vi "EditServerChannelInteractive.vi"() -> ()   [LabVIEW 2022 SP3]
uses:
  Sub VIs/ADAM Controls/Ch_description_ADAM.ctl
  Sub VIs/ADAM Controls/Module_type_ADAM.ctl
  Sub VIs/ADAM Controls/Function_ADAM.ctl
  Sub VIs/ADAM Controls/Channel_State.ctl
  Sub VIs/ADAM Controls/Calib_type_ADAM.ctl
  Sub VIs/ADAM Controls/Address.ctl
  Sub VIs/ADAM Controls/Channel_names.ctl
  EditServerChannelInteractive.ctl
  ADAM Server/ADAM_Global.vi
panel:
  in  "showFP":bool
  in  "chsOff":bool
  in  "chsOn":bool
  out "NewVal":i32[](array[numeric])
  in  "Set Value":dbl
  in  "channelTypes":T1
  in  "Channel Select":i32[](listbox)
  in  "stop":bool
  in  "reloadChannels":bool
  in  "deleteChannel":bool
  in  "reloadDescription":bool
  in  "updateChDescription":bool
  in  "updateValue":bool
  out "Message":string
  out "Value":dbl
  out "String":string
  out "Help":string
  in  "Search String":string
  in  "Ch Description":T2={"Ch Name"="", "Type"="", "Function"=enum."Analogue Input", "Ch State"=enum."On", "Calibration type"="", "A"=0.0, "B"=0.0, "C"=0.0, "D"=0.0, "Comments"="", "Address"={"Main"=0, "Ch."=0, "Sub"=0, "Port Name"=""}, "String"="", "Duty"=65535} {"Duty" format="%016b"; "D" format="%#_5g"; "C" format="%#_5g"; "B" format="%#_5g"; "A" format="%#_5g"}
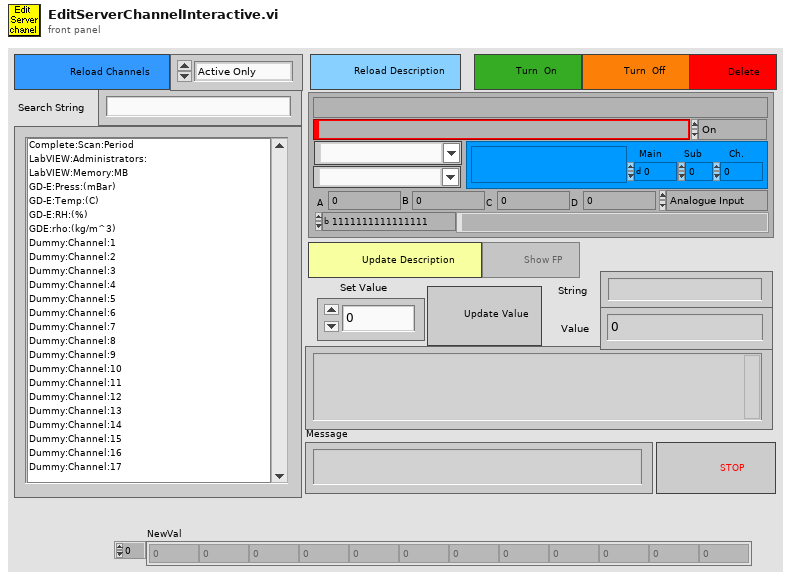
[diagram p1: front panel]
types:
  T1 = typedef "Channel_names.ctl" = enum16{"Active Only", "Active + Off", "All Channels", "Changeable Only", "Always Off", "Always On", "Always Off or On"}
  T2 = typedef "Ch_description_ADAM.ctl" = cluster{"Ch Name":string, "Type":T3, "Function":T4, "Ch State":T5, "Calibration type":T6, "A":dbl, "B":dbl, "C":dbl, "D":dbl, "Comments":string, "Address":T7, "String":string, "Duty":u16}
  T3 = typedef "Module_type_ADAM.ctl" = string
  T4 = typedef "Function_ADAM.ctl" = enum16{"Analogue Input", "Digital Input", "Event counter", "Event rate", "Analogue Output", "Digital Output", "Relay Output"}
  T5 = typedef "Channel_State.ctl" = enum16{"On", "Off", "Always On", "Always Off"}
  T6 = typedef "Calib_type_ADAM.ctl" = string
  T7 = typedef "Address.ctl" = cluster{"Main":i32, "Ch.":i32, "Sub":i32, "Port Name":string}
  T8 = typedef "EditServerChannelInteractive.ctl" = enum16{"Start", "Wait for user", "Check Channels", "Get Channel Names", "Get Current Value", "Get Channel Description", "Update Channel Value", "Update Channel State", "Update Channel Description", "Delete Channel", "Multi Channel", "openFP"}
  T9 = enum8{"Enabled", "Disabled", "Disabled and Grayed Out"}
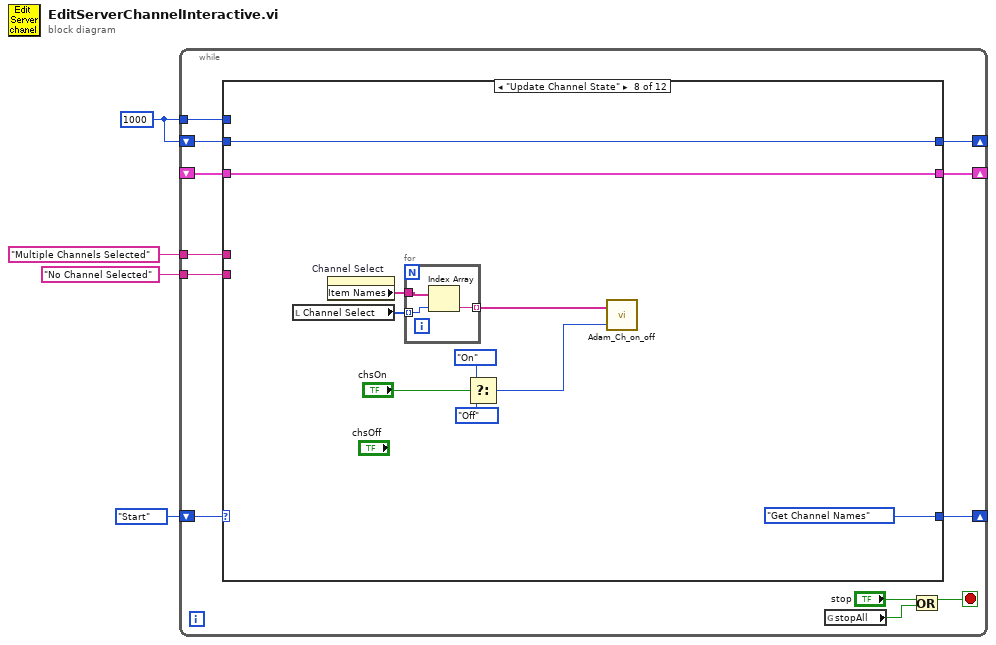
[diagram p0: block diagram]
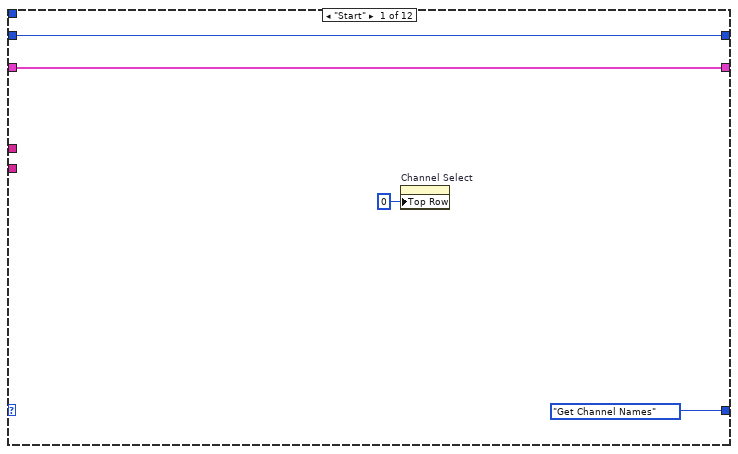
[diagram p2: hidden frame]
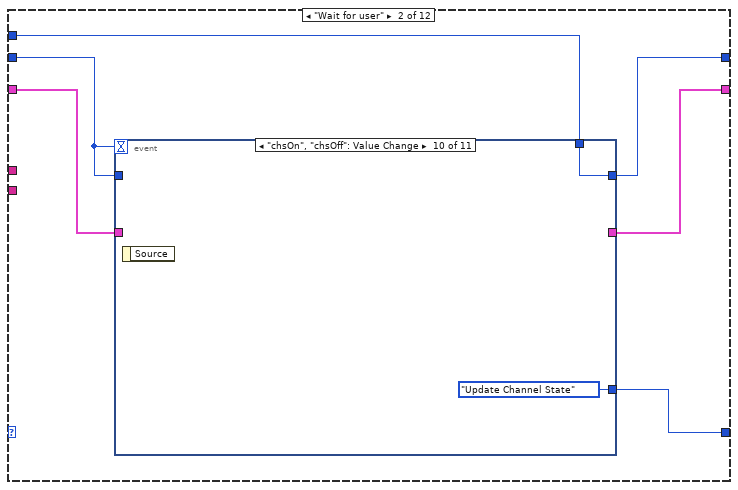
[diagram p3: hidden frame]
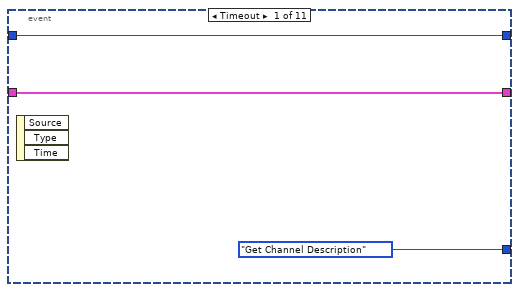
[diagram p4: hidden frame]
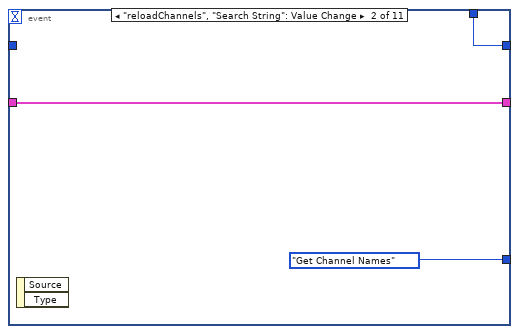
[diagram p5: hidden frame]
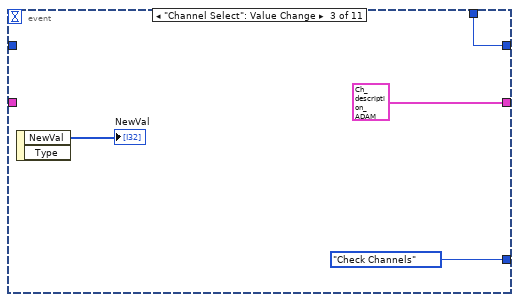
[diagram p6: hidden frame]
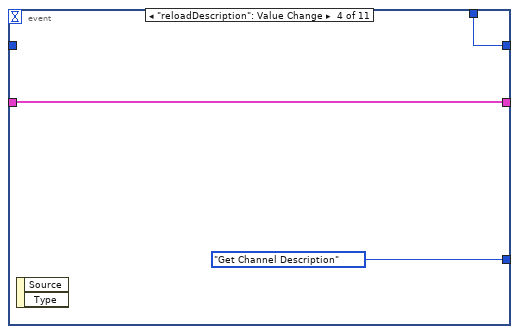
[diagram p7: hidden frame]
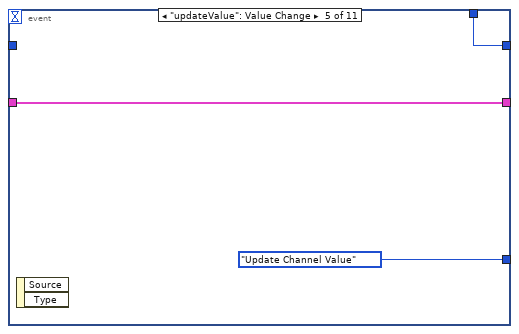
[diagram p8: hidden frame]
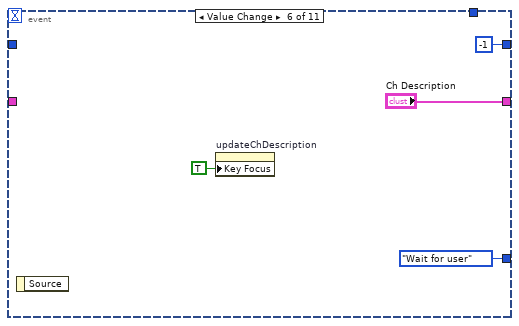
[diagram p9: hidden frame]
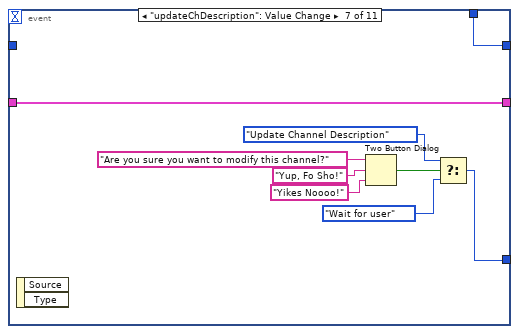
[diagram p10: hidden frame]
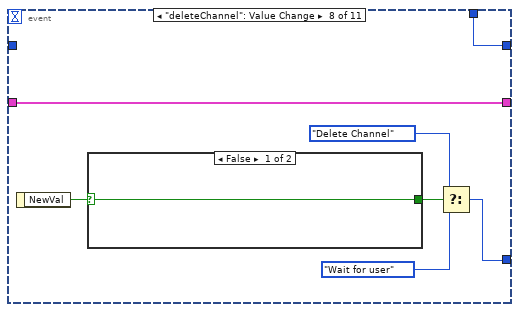
[diagram p11: hidden frame]
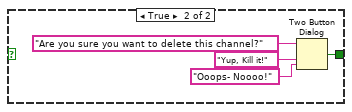
[diagram p12: hidden frame]
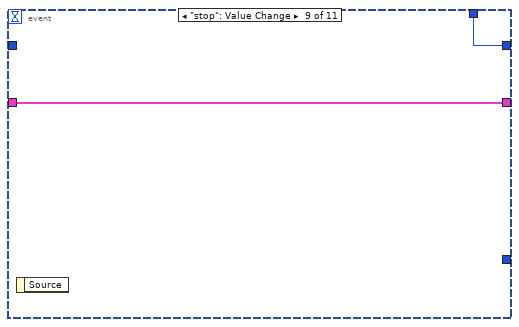
[diagram p13: hidden frame]
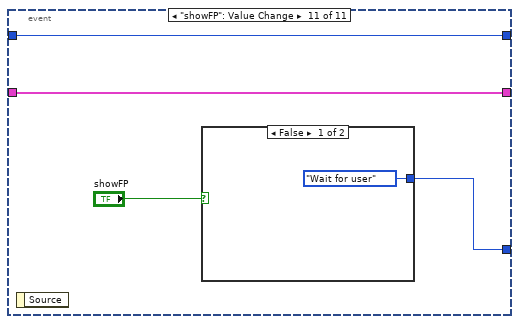
[diagram p14: hidden frame]
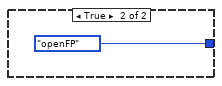
[diagram p15: hidden frame]
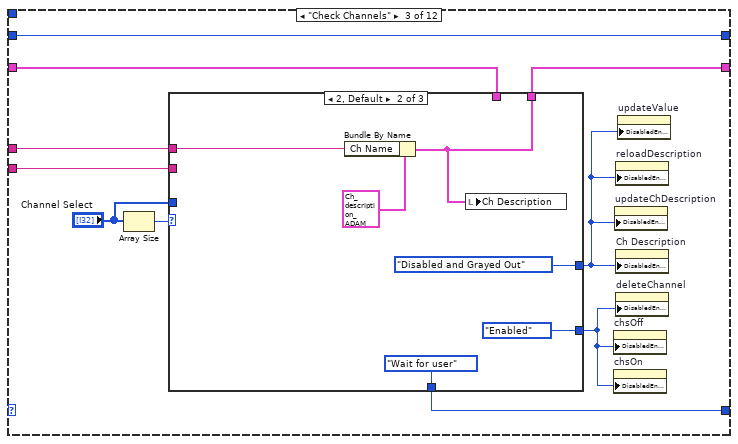
[diagram p16: hidden frame]
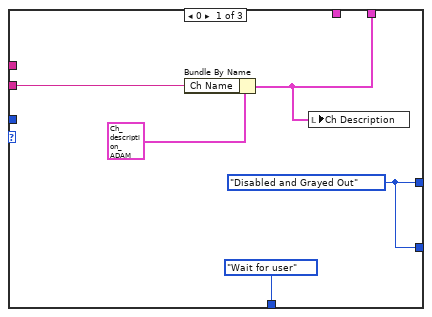
[diagram p17: hidden frame]
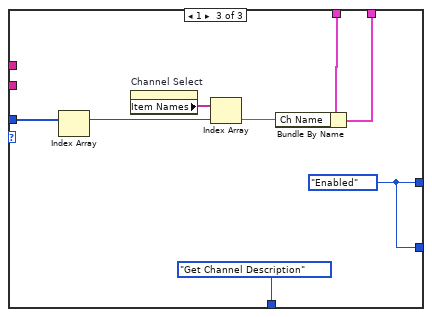
[diagram p18: hidden frame]
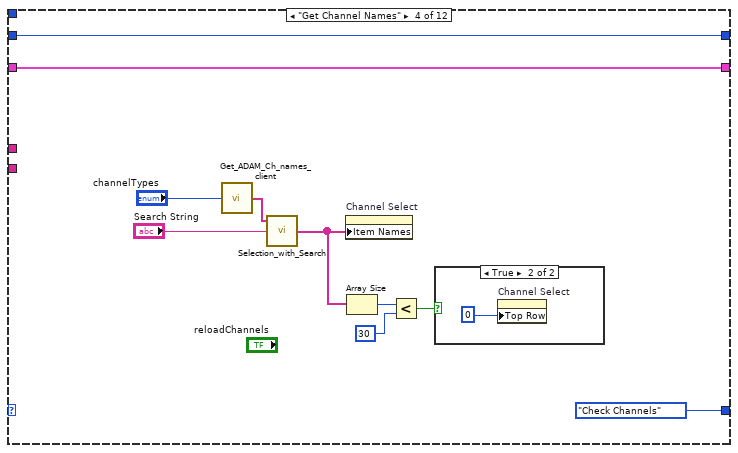
[diagram p19: hidden frame]
diagram:
  w1 = 1000
  n1 = while {
    shift-right: [w15] -> _
    shift-left: EditServerChannelInteractive."Start" ("Mode") -> [w16]
    shift-right: [w13] -> _
    shift-left: _ -> [w12]
    tunnel: "Multiple Channels Selected" ("Ch Name") -> [w11]
    tunnel: "No Channel Selected" ("Ch Name") -> [w10]
    shift-right: [w6] -> _
    shift-left: w1 -> [w7]
    tunnel: w1 -> [w5]
    stop <- w9 stop-if-true
    n2 = case shown="\"Update Channel State\"" w16 {
      tunnel: [EditServerChannelInteractive."Get Channel Names" ("Mode") w26 w85 EditServerChannelInteractive."Check Channels" ("Mode") EditServerChannelInteractive."Get Current Value" ("Mode") EditServerChannelInteractive."Wait for user" ("Mode") EditServerChannelInteractive."Get Current Value" ("Mode") EditServerChannelInteractive."Get Channel Names" ("Mode") EditServerChannelInteractive."Wait for user" ("Mode") EditServerChannelInteractive."Get Channel Names" ("Mode") EditServerChannelInteractive."Get Channel Names" ("Mode") EditServerChannelInteractive."Wait for user" ("Mode")] -> w15
      tunnel: [w19 w24 w82 w110 w120 w169 w185 w203 w208 w220 w235 w249] -> w13
      tunnel: w12 -> [w19 w25 w87 w110 w119 w169 w185 w203 w208 w220 w235 w249]
      tunnel: w11 -> [_ _ w84 _ _ _ _ _ _ _ _ _]
      tunnel: w10 -> [_ _ w81 _ _ _ _ _ _ _ _ _]
      tunnel: w7 -> [w17 w22 w78 w107 w118 w163 w183 w197 w212 w219 w230 w248]
      tunnel: [w17 w23 w78 w107 w118 w163 w183 w197 w212 w219 w230 w248] -> w6
      tunnel: w5 -> [_ w21 _ _ _ _ _ _ _ _ _ _]
      frame "Start" {
        n3 = property on="Channel Select" class="LstBox (strict)"("Top Row"=0) -> ()  [unwired: 2 in, 2 out]
      }
      frame "Wait for user" {
        n4 = event shown="[9] \"chsOn\", \"chsOff\": Value Change" {
          selector: _ -> [_ _ _ _ _ _ _ _ _ _ _]
          dyn-events: _ -> [_ _ _ _ _ _ _ _ _ _ _]
          timeout: w22 -> [_ _ _ _ _ _ _ _ _ _ _]
          tunnel: [EditServerChannelInteractive."Get Channel Description" ("Mode") EditServerChannelInteractive."Get Channel Names" ("Mode") EditServerChannelInteractive."Check Channels" ("Mode") EditServerChannelInteractive."Get Channel Description" ("Mode") EditServerChannelInteractive."Update Channel Value" ("Mode") EditServerChannelInteractive."Wait for user" ("Mode") w48 w60 _ EditServerChannelInteractive."Update Channel State" ("Mode") w74] -> w26
          tunnel: [w28 w31 T2 {"Ch Name"="", "Type"="", "Function"=enum."Analogue Input", "Ch State"=enum."On", "Calibration type"="", "A"=0.0, "B"=0.0, "C"=0.0, "D"=0.0, "Comments"="", "Address"={"Main"=0, "Ch."=0, "Sub"=0, "Port Name"=""}, "String"="", "Duty"=65535} ("Ch Description") w38 w41 "Ch Description" w55 w62 w69 _ w72] -> w24
          tunnel: w25 -> [w28 w31 _ w38 w41 _ w55 w62 w69 _ w72]
          tunnel: [w27 w30 w33 w37 w40 -1 w47 w56 w68 w70 w75] -> w23
          tunnel: w22 -> [w27 _ _ _ _ _ _ _ _ _ w75]
          tunnel: w21 -> [_ w30 w33 w37 w40 _ w47 w56 w68 w70 _]
          event Timeout {
            n5 = event-data() -> ()  [unwired: 1 in, 3 out]
          }
          event "reloadChannels", "Search String": Value Change {
            n6 = event-data() -> ()  [unwired: 1 in, 2 out]
          }
          event "Channel Select": Value Change {
            n7 = event-data() -> ("NewVal"=→"NewVal":i32[])  [unwired: 1 in, 1 out]
          }
          event "reloadDescription": Value Change {
            n8 = event-data() -> ()  [unwired: 1 in, 2 out]
          }
          event "updateValue": Value Change {
            n9 = event-data() -> ()  [unwired: 1 in, 2 out]
          }
          event Value Change {
            n10 = event-data() -> ()  [unwired: 1 in, 1 out]
            n11 = property on="updateChDescription" class="Bool"("Key Focus"=TRUE) -> ()  [unwired: 2 in, 2 out]
          }
          event "updateChDescription": Value Change {
            n12 = event-data() -> ()  [unwired: 1 in, 2 out]
            n13 = Two Button Dialog(message="Are you sure you want to modify this channel?", 1:"Yikes Noooo!" ("F button name (\"Cancel\")"), 2:"Yup, Fo Sho!" ("T button name (\"OK\")")) -> (T button?=w54:bool)
            n14 = Select(t=EditServerChannelInteractive."Update Channel Description" ("Mode"), s=w54, f=EditServerChannelInteractive."Wait for user" ("Mode")) -> (s? t:f=w48:T8)
          }
          event "deleteChannel": Value Change {
            n15 = event-data() -> ("NewVal"=w57:bool)  [unwired: 1 in]
            n16 = case shown="False" w57 {
              selector: w57 -> [w63 _]
              tunnel: [w63 w64] -> w61
              frame False {
              }
              frame True {
                n17 = Two Button Dialog(message="Are you sure you want to delete this channel?", 1:"Ooops- Noooo!" ("F button name (\"Cancel\")"), 2:"Yup, Kill it!" ("T button name (\"OK\")")) -> (T button?=w64:bool)
              }
            }
            n18 = Select(t=EditServerChannelInteractive."Delete Channel" ("Mode"), s=w61, f=EditServerChannelInteractive."Wait for user" ("Mode")) -> (s? t:f=w60:T8)
          }
          event "stop": Value Change {
            n19 = event-data() -> ()  [unwired: 1 in, 1 out]
          }
          event "chsOn", "chsOff": Value Change {
            n20 = event-data() -> ()  [unwired: 1 in, 1 out]
          }
          event "showFP": Value Change {
            n21 = event-data() -> ()  [unwired: 1 in, 1 out]
            n22 = case shown="False" "showFP" {
              tunnel: [EditServerChannelInteractive."Wait for user" ("Mode") EditServerChannelInteractive."openFP" ("Mode")] -> w74
              frame False {
              }
              frame True {
              }
            }
          }
        }
      }
      frame "Check Channels" {
        n23 = Array Size(array="Channel Select") -> (size(s)=w86:i32)
        n24 = case shown="2, Default" w86 {
          tunnel: w87 -> [_ _ w104]
          tunnel: [w90 w94 w103] -> w82
          tunnel: [EditServerChannelInteractive."Wait for user" ("Mode") EditServerChannelInteractive."Wait for user" ("Mode") EditServerChannelInteractive."Get Channel Description" ("Mode")] -> w85
          tunnel: [w88 T9."Disabled and Grayed Out" ("Disabled") w99] -> w80
          tunnel: w84 -> [_ w95 _]
          tunnel: "Channel Select" -> [_ _ w101]
          tunnel: w81 -> [w89 _ _]
          tunnel: [w88 T9."Enabled" ("Disabled") w99] -> w79
          frame 0 {
            w88 = T9."Disabled and Grayed Out" ("Disabled")
            n25 = Bundle By Name(cluster=T2 {"Ch Name"="", "Type"="", "Function"=enum."Analogue Input", "Ch State"=enum."On", "Calibration type"="", "A"=0.0, "B"=0.0, "C"=0.0, "D"=0.0, "Comments"="", "Address"={"Main"=0, "Ch."=0, "Sub"=0, "Port Name"=""}, "String"="", "Duty"=65535} ("Ch Discription"), "Ch Name"=w89) -> (w90:T2)
            n26 = local write "Ch Description"(w90) -> ()
          }
          frame 2, Default {
            n27 = Bundle By Name(cluster=T2 {"Ch Name"="", "Type"="", "Function"=enum."Analogue Input", "Ch State"=enum."On", "Calibration type"="", "A"=0.0, "B"=0.0, "C"=0.0, "D"=0.0, "Comments"="", "Address"={"Main"=0, "Ch."=0, "Sub"=0, "Port Name"=""}, "String"="", "Duty"=65535} ("Ch Discription"), "Ch Name"=w95) -> (w94:T2)
            n28 = local write "Ch Description"(w94) -> ()
          }
          frame 1 {
            w99 = T9."Enabled" ("Disabled")
            n29 = Index Array(array=w101) -> (element=w100:i32)  [unwired: 1 in]
            n30 = property on="Channel Select" class="LstBox (strict)"() -> ("Item Names"=w105:string[])  [unwired: 2 in, 2 out]
            n31 = Index Array(array=w105, index=w100) -> (element=w106:string)
            n32 = Bundle By Name(cluster=w104, "Ch Name"=w106) -> (w103:T2)
          }
        }
        n33 = property on="chsOff" class="Bool"("DisabledEnum"=w79) -> ()  [unwired: 2 in, 2 out]
        n34 = property on="chsOn" class="Bool"("DisabledEnum"=w79) -> ()  [unwired: 2 in, 2 out]
        n35 = property on="updateChDescription" class="Bool"("DisabledEnum"=w80) -> ()  [unwired: 2 in, 2 out]
        n36 = property on="reloadDescription" class="Bool"("DisabledEnum"=w80) -> ()  [unwired: 2 in, 2 out]
        n37 = property on="Ch Description" class="Clust (strict)"("DisabledEnum"=w80) -> ()  [unwired: 2 in, 2 out]
        n38 = property on="deleteChannel" class="Bool"("DisabledEnum"=w79) -> ()  [unwired: 2 in, 2 out]
        n39 = property on="updateValue" class="Bool"("DisabledEnum"=w80) -> ()  [unwired: 2 in, 2 out]
      }
      frame "Get Channel Names" {
        n40 = call "Get_ADAM_Ch_names_client.vi"("Channel names set"="channelTypes") -> ("Ch names"=w116:string[])
        n41 = call "Selection_with_Search.vi"("Search String"="Search String", "All Channel Names"=w116) -> ("Item Names"=w109:string[])  [unwired: 1 in]
        n42 = property on="Channel Select" class="LstBox (strict)"("Item Names"=w109) -> ()  [unwired: 2 in, 2 out]
        n43 = Array Size(array=w109) -> (size(s)=w115:i32)
        n44 = Less?(x=w115, y=30) -> (x < y?=w113:bool)
        n45 = case shown="True" w113 {
          frame False {
          }
          frame True {
            n46 = property on="Channel Select" class="LstBox (strict)"("Top Row"=0) -> ()  [unwired: 2 in, 2 out]
          }
        }
      }
      frame "Get Channel Description" {
        # "#ToDo Use DoADAMChannel, so all types are automatically available"
        n47 = Unbundle By Name(w119) -> ("Ch Name"=w121:string)
        n48 = call "Get_Current_Scan_client.vi"("singleChannel"=w121) -> ("Ch Description Array"=w125:T2[], "String values"=w124:string[], "Numerical Values"=w123:dbl[])  [unwired: 1 in, 1 out]
        n49 = for {
          tunnel: w125 -> [w128] mode=indexing
          tunnel: w124 -> [w129] mode=indexing
          tunnel: w123 -> [w130] mode=indexing
          tunnel: [w128] -> w120
          n50 = Unbundle By Name(w128) -> ("Function"=w131:T4, "Type"=w135:T3)
          n51 = Bundle By Name(cluster=w128, "Type"=T3 "Help") -> (w133:T2)
          n52 = local write "String"(w129) -> ()
          n53 = local write "Value"(w130) -> ()
          n54 = case shown="\"ScanPacer\"" w135 {
            tunnel: ["Sorry; help not available for this channel type" w139 "Value A is the default reset time value in seconds" w145 w146 "\"A\" is the max RPM that can be set" w149 w151 w154 w157 w159 w161] -> w132
            tunnel: w133 -> [_ _ _ w144 w147 _ w150 w152 w156 w158 w160 w162]
            tunnel: w131 -> [_ w140 _ _ _ _ _ _ _ _ _ _]
            frame "4011", Default {
            }
            frame "TENMA 72-2xxx" {
              n55 = case shown="\"Analogue Input\", Default" w140 {
                tunnel: ["Sorry; help not available" "A is \"Initial current limit (A)\"\nB is \"Running current limit (A)\"\nC is \"Initial wait (ms)\""] -> w139
                frame "Analogue Input", Default {
                }
                frame "Analogue Output" {
                }
              }
            }
            frame "Count Down Timer" {
            }
            frame "Comparator" {
              n56 = call "Comparator.vi"("Ch Description"=w144) -> ("HelpText"=w145:string)  [unwired: 6 in, 2 out]
            }
            frame "Average", "St Deviation" {
              n57 = call "Stats.vi"("Ch Description"=w147) -> ("HelpText"=w146:string)  [unwired: 6 in, 2 out]
            }
            frame "Set Motor RPM" {
            }
            frame "AutoZero" {
              n58 = call "CPP-ZeroMonitor.vi"("Ch Description"=w150) -> ("HelpText"=w149:string)  [unwired: 6 in, 2 out]
            }
            frame "Equation" {
              n59 = call "CPP-Equation.vi"("Ch Description"=w152) -> ("HelpText"=w151:string)  [unwired: 6 in, 2 out]
            }
            frame "ScanPacer" {
              n60 = call "ADAMPacer.vi"("Ch Description"=w156) -> ("HelpText"=w155:string)  [unwired: 6 in, 2 out]
              n61 = Concatenate Strings(w155, "\nNote: not required if you use Minimum Scan Period (ms) in Scan_mode.txt " ("string")) -> (w154:string)
            }
            frame "DLI WebPowerSwitch" {
              n62 = call "DLIWebPowerSwitch.vi"("Ch Description"=w158) -> ("HelpText"=w157:string)  [unwired: 6 in, 2 out]
            }
            frame "AalborgMFC" {
              n63 = call "AalborgMFC.vi"("Ch Description"=w160) -> ("HelpText"=w159:string)  [unwired: 6 in, 2 out]
            }
            frame "AlicatMFC" {
              n64 = call "AlicatMFC.vi"("Ch Description"=w162) -> ("HelpText"=w161:string)  [unwired: 6 in, 2 out]
            }
          }
          "Help" <- w132
          n65 = Unbundle By Name(w128) -> ("Type"=w127:T3)
          n66 = local write "Ch Description"(w128) -> ()
          n67 = case shown="\"False\", Default" w127 {
            tunnel: [T9."Disabled and Grayed Out" ("Disabled") T9."Enabled" ("Disabled")] -> w126
            frame "False", Default {
            }
            frame "Run VI Named:" {
            }
          }
          n68 = property on="showFP" class="Bool"("DisabledEnum"=w126) -> ()  [unwired: 2 in, 2 out]
        }
      }
      frame "Get Current Value" {
        n69 = Unbundle By Name(w169) -> ("Calibration type"=w164:T6, "Ch Name"=w170:string)
        n70 = call "Get_Current_Scan_client.vi"("singleChannel"=w170) -> ("Ch Description Array"=w165:T2[], "String values"=w168:string[], "Numerical Values"=w167:dbl[])  [unwired: 1 in, 1 out]
        n71 = for {
          tunnel: w168 -> [w172] mode=indexing
          tunnel: w167 -> [w171] mode=indexing
          tunnel: w165 -> [w175] mode=indexing
          tunnel: w164 -> [w174]
          n72 = case shown="\"Text\"" w174 {
            tunnel: w175 -> [_ w182]
            tunnel: [w176 w177] -> w173
            tunnel: w172 -> [w176 _]
            tunnel: w171 -> [_ w178]
            frame "False", Default {
            }
            frame "Text" {
              n73 = Unbundle By Name(w182) -> ("String"=w181:string)
              n74 = call <vilib>:"Delimited String to 1D String Array.vi"("delimiter"=";", "delimited string"=w181) -> ("string array"=w179:string[])  [unwired: 9 in]
              n75 = Index Array(array=w179, index=w178) -> (element=w177:string)
            }
          }
          "String" <- w173
          "Value" <- w171
        }
      }
      frame "Update Channel Value" {
        n76 = Unbundle By Name(w185) -> ("Ch Name"=w186:string)
        n77 = Build Array("Set Value") -> (w191:dbl[])
        n78 = Build Array(w186) -> (w192:string[])
        n79 = call "ASYNC_Adam_client.vi"("Values"=w191, "Channel Names"=w192) -> ("Scan Comments"=w188:string[], "Calibrated Units"=w189:dbl[])  [unwired: 1 in]
        n80 = for {
          N: 1 -> [_]
          tunnel: w189 -> [w194] mode=indexing
          tunnel: w188 -> [w193] mode=indexing
          n81 = local write "Value"(w194) -> ()
          "Message" <- w193
        }
      }
      frame "Update Channel State" {
        n82 = local read "Channel Select"() -> (w201:i32[])
        n83 = property on="Channel Select" class="LstBox (strict)"() -> ("Item Names"=w202:string[])  [unwired: 2 in, 2 out]
        n84 = for {
          tunnel: w202 -> [w207]
          tunnel: w201 -> [w206] mode=indexing
          tunnel: [w205] -> w196 mode=indexing
          n85 = Index Array(array=w207, index=w206) -> (element=w205:string)
        }
        n86 = Select(t=Channel_State."On" ("Ch State"), s="chsOn", f=Channel_State."Off" ("Ch State")) -> (s? t:f=w195:T5)
        n87 = call "Adam_Ch_on_off.vi"("Ch State"=w195, "ADAM Ch Names"=w196) -> ()  [unwired: 1 out]
      }
      frame "openFP" {
        n88 = Unbundle By Name(w208) -> ("Type"=w209:T3, "Comments"=w210:string)
        n89 = case shown="\"Run VI Named:\"" w209 {
          tunnel: w210 -> [_ w218]
          frame "False", Default {
            n90 = One Button Dialog(message="Sorry- can currently only open RunVI Named channels") -> ()  [unwired: 1 in, 1 out]
          }
          frame "Run VI Named:" {
            n91 = Current VI's Path() -> (path=w216:path)
            n92 = Build Path(base path=w216, name or relative path=path "../../../ADAM Server/Run_vi_named" ("base path")) -> (appended path=w214:path)
            n93 = Build Path(base path=w214, name or relative path=w218) -> (appended path=w217:path)
            n94 = call "Open_Close_Front_Panel.ph.vi"("VI path"=w217) -> ()  [unwired: 2 in, 1 out]
          }
        }
      }
      frame "Update Channel Description" {
        n95 = Unbundle By Name(w220) -> ("Ch Name"=w226:string)
        n96 = call "Check_Ch_Name_colons.vi"("No of Colons"=2, "Ch Name in"=w226) -> ("Ch Name out"=w224:string)
        n97 = Bundle By Name(cluster=w220, "Ch Name"=w224) -> (w223:T2)
        n98 = Empty String/Path?(string/path=w226) -> (empty?=w222:bool)
        n99 = case shown="False" w222 {
          tunnel: w223 -> [w228 _]
          frame False {
            n100 = Build Array(w228) -> (w229:T2[])
            n101 = call "Update_Ch_Discription_client.vi"("Channels to update In"=w229) -> ()  [unwired: 1 out]
            n102 = Wait (ms)(milliseconds to wait=u32 1100) -> ()  [unwired: 1 out]
          }
          frame True {
          }
        }
      }
      frame "Delete Channel" {
        w234 = T2 {"Ch Name"="", "Type"="", "Function"=enum."Analogue Input", "Ch State"=enum."On", "Calibration type"="", "A"=0.0, "B"=0.0, "C"=0.0, "D"=0.0, "Comments"="", "Address"={"Main"=0, "Ch."=0, "Sub"=0, "Port Name"=""}, "String"="", "Duty"=0}  # Ch Discription
        n103 = local read "Channel Select"() -> (w237:i32[])
        n104 = property on="Channel Select" class="LstBox (strict)"() -> ("Item Names"=w236:string[])  [unwired: 2 in, 2 out]
        n105 = for {
          tunnel: w237 -> [w247] mode=indexing
          tunnel: w236 -> [w246]
          tunnel: [w244] -> w233 mode=indexing
          tunnel: w234 -> [w242]
          n106 = Index Array(array=w246, index=w247) -> (element=w245:string)
          n107 = Bundle By Name(cluster=w242, "Ch Name"=w245, "Address.Port Name"="DELETE" ("Comments")) -> (w244:T2)
        }
        n108 = Array Size(array=w233) -> (size(s)=w232:i32)
        n109 = case shown="1, Default" w232 {
          tunnel: w233 -> [w240 _]
          tunnel: [u32 1100 ("milliseconds to wait") u32 0 ("milliseconds to wait")] -> w231
          frame 1, Default {
            n110 = call "Update_Ch_Discription_client.vi"("Channels to update In"=w240) -> ()  [unwired: 1 out]
          }
          frame 0 {
          }
        }
        n111 = Wait (ms)(milliseconds to wait=w231) -> ()  [unwired: 1 out]
      }
      frame "Multi Channel" {
      }
    }
    n112 = global read "ADAM_Global.vi" "stopAll"() -> (w8:bool)
    n113 = Or(x="stop", y=w8) -> (x .or. y?=w9:bool)
  }
